vi "Hanning Window.vi"   [LabVIEW 2010, in "NI_AALPro.lvlib"]
doc: "Applies a Hanning window to the input signal <B>X</B>. Wire data to the <B>X</B> input to determine the polymorphic instance to use or manually select the instance."
uses:
  NI_AALPro.lvlib
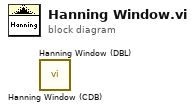
[diagram p0: block diagram]
diagram:
  n1 = call "Hanning Window (CDB).vi"() -> ()  [unwired: 1 in, 2 out]
  n2 = call "Hanning Window (DBL).vi"() -> ()  [unwired: 1 in, 2 out]
